vi "New result.vi"(8 "error in (no error)":errorcluster, 10 "Result":refnum<class "Mag Lab Result.lvclass">, 11 "Settle Output in":refnum<class "Settle Output.lvclass">) -> (0 "error out":errorcluster, 2 "Is output settled?":bool, 3 "Settle Output out":refnum<class "Settle Output.lvclass">)   [LabVIEW 2015, in "Settle Output.lvclass"]
uses:
  Settle Output.lvclass
  Mag Lab Result/Mag Lab Result.lvclass
  Mag Lab Result/DBL Result/DBL Result.lvclass
  Settle Output.lvclass/Settle Output.ctl
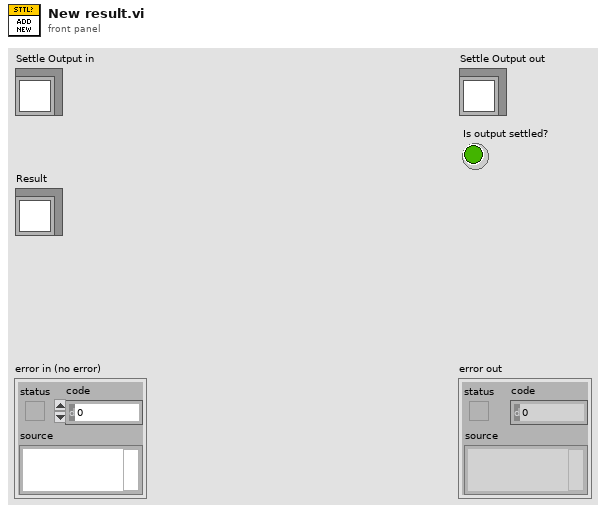
[diagram p1: front panel]
types:
  T1 = cluster{"seconds since 1Jan1904":timestamp, "Value":dbl}
  T2 = cluster{"seconds since 1Jan1904":timestamp, "Value":dbl}[]
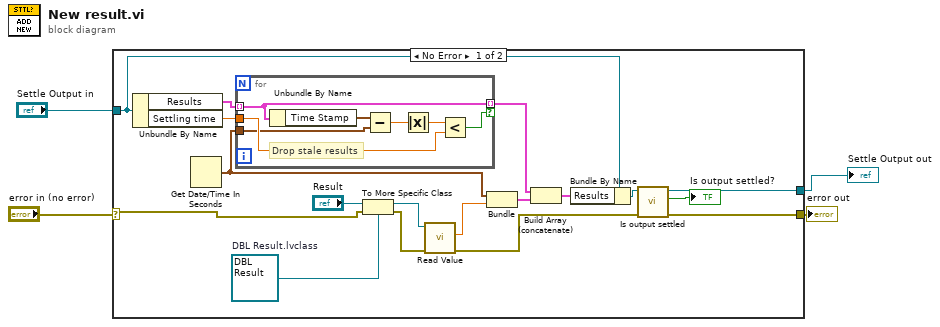
[diagram p0: block diagram]
diagram:
  n1 = case shown="No Error" "error in (no error)" {
    selector: "error in (no error)" -> [w9 w31]
    tunnel: [w12 w31] -> w3
    tunnel: [w13 w30] -> w1
    tunnel: "Settle Output in" -> [w22 w30]
    frame No Error {
      w10 = refnum<class "DBL Result.lvclass"> refnum  # DBL Result.lvclass
      n2 = Unbundle By Name(w22) -> ("Results"=w21:cluster{"Time Stamp":timestamp, "Result":dbl}[], "Settling time"=w20:dbl)
      n3 = Get Date/Time In Seconds() -> (seconds since 1Jan1904=w18:timestamp)
      n4 = for {
        tunnel: w21 -> [w27] mode=indexing
        tunnel: w18 -> [w24]
        tunnel: w20 -> [w28]
        tunnel: [w27] -> w19 mode=indexing if=w26
        # "Drop stale results"
        n5 = Unbundle By Name(w27) -> ("Time Stamp"=w25:timestamp)
        n6 = Subtract(x=w25, y=w24) -> (x-y=w29:dbl)
        n7 = Absolute Value(x=w29) -> (abs(x)=w23:dbl)
        n8 = Less?(x=w23, y=w28) -> (x < y?=w26:bool)
      }
      n9 = To More Specific Class(target class=w10, reference="Result", error in=w9) -> (specific class reference=w8:refnum<class "DBL Result.lvclass">, error out=w7:errorcluster)
      n10 = call-dynamic "Read Value.vi"("error in (no error)"=w7, "DBL Result in"=w8) -> ("error out"=w5:errorcluster, "Value"=w6:dbl)  [unwired: 7 in, 1 out]
      n11 = Bundle("seconds since 1Jan1904"=w18, "Value"=w6) -> (w16:T1)  [unwired: 1 in]
      n12 = Build Array (concatenate)(w19, w16) -> (w15:T2)
      n13 = Bundle By Name(cluster=w22, "Results"=w15) -> (w14:refnum<class "Settle Output.lvclass">)
      n14 = call-dynamic "Is output settled.vi"("error in (no error)"=w5, "Settle Output in"=w14) -> ("error out"=w12:errorcluster, "Is output settled?"=→"Is output settled?":bool, "Settle Output out"=w13:refnum<class "Settle Output.lvclass">)  [unwired: 7 in]
    }
    frame Error {
    }
  }
  "error out" <- w3
  "Settle Output out" <- w1
